vi "Read Stream.vi"(8 "error in (no error)":errorcluster, 11 "SECS-II Class in":refnum<class "SECS-II Class.lvclass">) -> (0 "error out":errorcluster, 2 "Stream":u8, 3 "SECS-II Class out":refnum<class "SECS-II Class.lvclass">)   [LabVIEW 2020, in "SECS Communication.lvlib" / "SECS-II Class.lvclass"]
uses:
  SECS-II Class.lvclass
  SECS-II Class.lvclass/SECS-II Class.ctl
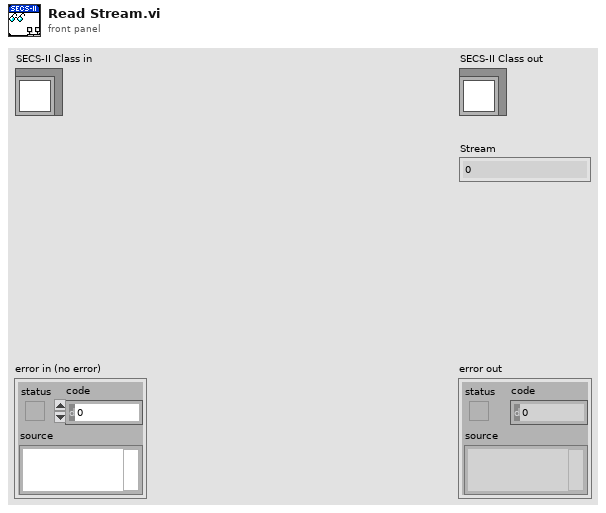
[diagram p1: front panel]
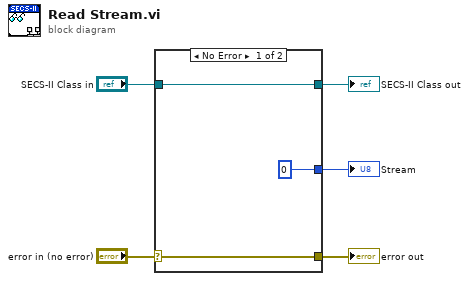
[diagram p0: block diagram]
diagram:
  n1 = case shown="No Error" "error in (no error)" {
    selector: "error in (no error)" -> [w8 w9]
    tunnel: [w8 w9] -> w4
    tunnel: [w7 w10] -> w2
    tunnel: "SECS-II Class in" -> [w7 w10]
    tunnel: [u8 0 _] -> w1
    frame No Error {
    }
    frame Error {
    }
  }
  "error out" <- w4
  "SECS-II Class out" <- w2
  "Stream" <- w1
